vi "elapsedSamplingSecondsModule.vi"(7 "Command":T1, 8 "error in (no error)":errorcluster, 10 "Time In":dbl) -> (0 "error out":errorcluster, 1 "Elapsed Out":dbl, 2 "Time Elapsed":bool)   [LabVIEW 2017]
uses:
  Timing_Module Control.ctl
panel:
  # "Input Data"
  # "Local Data"
  # "Output Data"
  # "No Local Data"
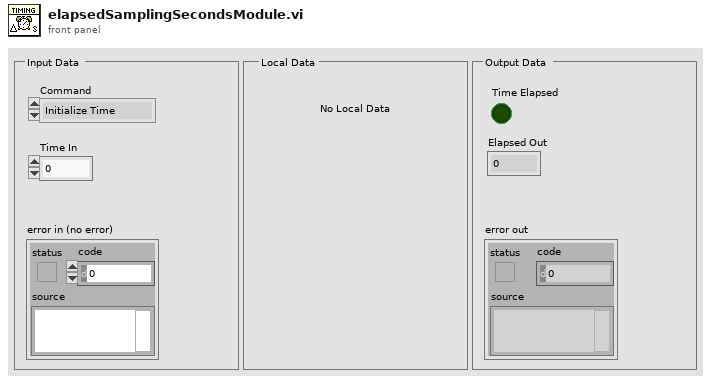
[diagram p1: front panel]
types:
  T1 = typedef "Timing_Module Control.ctl" = enum16{"Initialize Time", "Check Time"}
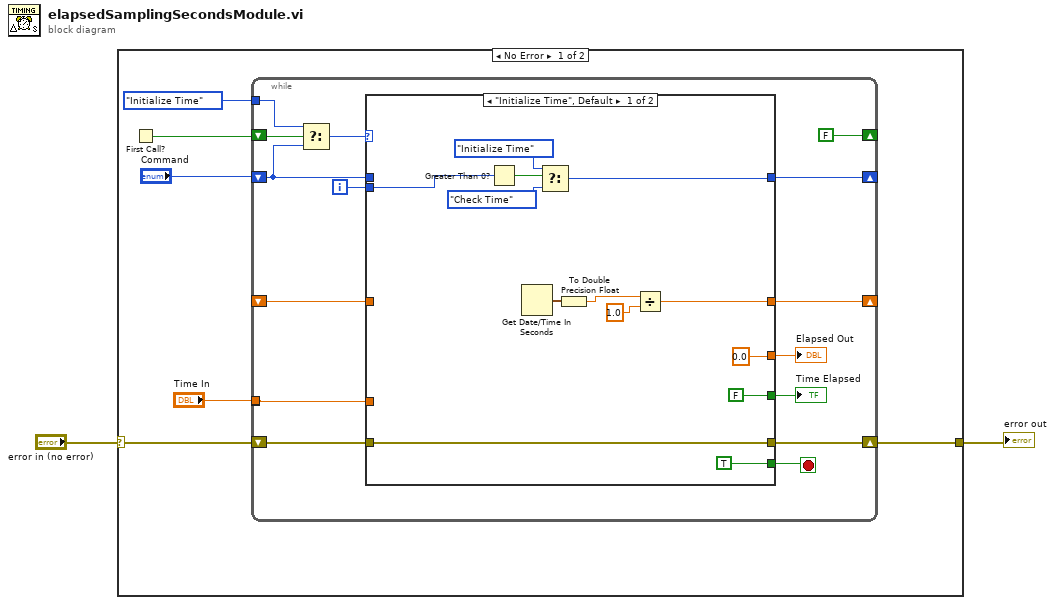
[diagram p0: block diagram]
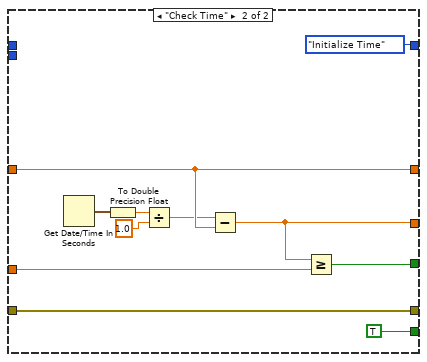
[diagram p2: hidden frame]
diagram:
  n1 = case shown="No Error" "error in (no error)" {
    selector: "error in (no error)" -> [w6 w48]
    tunnel: [w5 w48] -> w1
    frame No Error {
      n2 = First Call?() -> (First Call?: T/F=w8:bool)
      n3 = while {
        shift-right: [w15] -> _
        shift-left: "Command" -> [w16]
        shift-right: [w18] -> w5
        shift-left: w6 -> [w19]
        shift-right: [FALSE ("First Call?: T/F")] -> _
        shift-left: w8 -> [w23]
        tunnel: Timing_Module_Control."Initialize Time" ("t") -> [w22]
        shift-right: [w13] -> _
        shift-left: _ -> [w10]
        tunnel: [w9] -> _
        tunnel: "Time In" -> [w9]
        i -> [w14]
        stop <- w20 stop-if-true
        n4 = Select(t=w22, s=w23, f=w16) -> (s? t:f=w21:T1)
        n5 = case shown="\"Initialize Time\", Default" w21 {
          tunnel: [TRUE TRUE] -> w20
          tunnel: w19 -> [w35 w47]
          tunnel: [w35 w47] -> w18
          tunnel: w16 -> [_ _]
          tunnel: [w34 Timing_Module_Control."Initialize Time" ("t")] -> w15
          tunnel: w14 -> [w32 _]
          tunnel: [w26 w43] -> w13
          tunnel: [0.0 w42] -> w12
          tunnel: [FALSE w40] -> w11
          tunnel: w10 -> [_ w43]
          tunnel: w9 -> [_ w41]
          frame "Initialize Time", Default {
            n6 = Greater Than 0?(x=w32) -> (x > 0?=w31:bool)
            n7 = Get Date/Time In Seconds() -> (seconds since 1Jan1904=w29:timestamp)
            n8 = Select(t=Timing_Module_Control."Initialize Time", s=w31, f=Timing_Module_Control."Check Time" ("t")) -> (s? t:f=w34:T1)
            n9 = To Double Precision Float(number=w29) -> (double precision float=w25:dbl)
            n10 = Divide(x=w25, y=1.0) -> (x/y=w26:dbl)
          }
          frame "Check Time" {
            n11 = Get Date/Time In Seconds() -> (seconds since 1Jan1904=w44:timestamp)
            n12 = To Double Precision Float(number=w44) -> (double precision float=w38:dbl)
            n13 = Divide(x=w38, y=1.0) -> (x/y=w37:dbl)
            n14 = Subtract(x=w37, y=w43) -> (x-y=w42:dbl)
            n15 = Greater Or Equal?(x=w42, y=w41) -> (x >= y?=w40:bool)
          }
        }
        "Elapsed Out" <- w12
        "Time Elapsed" <- w11
      }
    }
    frame Error {
    }
  }
  "error out" <- w1
